vi "Initialise Notifiers and Ques.vi"(8 "error in (no error)":errorcluster) -> (0 "error out":errorcluster, 2 "Logging Queue out":refnum<queue>, 3 "Notifiers":T1)   [LabVIEW 2020]
uses:
  _Controls/Notifiers.ctl
  _Controls/Logging Queue Cluster.ctl
  _Controls/Tweezertron Ctrl Refs.ctl
  _Controls/Confocal Controls.ctl
  _Controls/iFlex.ctl
  _Controls/PIFOC Position.ctl
  _Controls/Manlight Controls.ctl
  _Controls/Exp Params.ctl
  _Controls/Image Thresholds.ctl
  _Controls/Spots.ctl
  _Controls/Spot Params.ctl
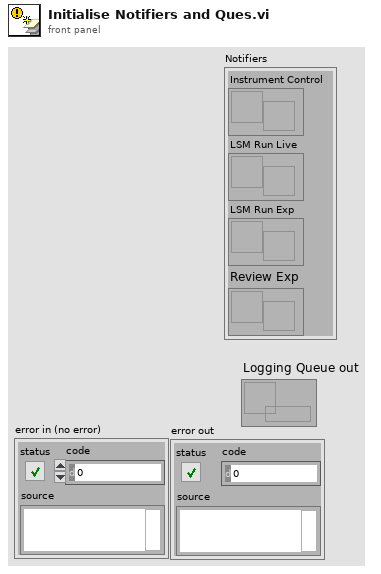
[diagram p1: front panel]
types:
  T1 = typedef "Notifiers.ctl" = cluster{"Instrument Control":refnum<notifier>, "LSM Run Live":refnum<notifier>, "LSM Run Exp":refnum<notifier>, "Review Exp":refnum<notifier>}
  T2 = typedef "Logging Queue Cluster.ctl" = cluster{"message":string, "Data for Logging":cluster{"pDataBuffer":u16[], "timestamp (ns)":u64, "PI pos (um)":dbl}, "Tweezertron Ctrl Refs":T3}
  T3 = typedef "Tweezertron Ctrl Refs.ctl" = cluster{"LSM Settings":refnum<vi>, "iFlex Control":refnum<vi>, "PIFOC Settings":refnum<vi>, "PinSelector":refnum<vi>, "Manlight Controls":refnum<vi>, "Exp Params":refnum<vi>, "Image Thresholds":refnum<vi>, "RevFrame":refnum<vi>, "Spots":refnum<vi>}
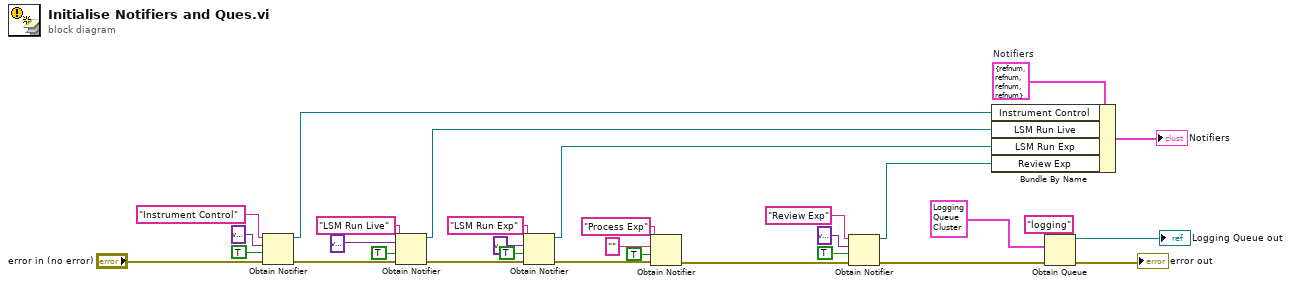
[diagram p0: block diagram]
diagram:
  w31 = T1 {"Instrument Control"=refnum, "LSM Run Live"=refnum, "LSM Run Exp"=refnum, "Review Exp"=refnum}  # Notifiers
  n1 = Obtain Notifier(name (unnamed)="Instrument Control", notification data type=variant ("element data type"), create if not found? (T)=TRUE, error in (no error)="error in (no error)") -> (notifier out=w16:refnum<notifier>, error out=w14:errorcluster)  [unwired: 1 out]
  n2 = Obtain Notifier(name (unnamed)="LSM Run Live", notification data type=variant ("element data type"), create if not found? (T)=TRUE, error in (no error)=w14) -> (notifier out=w28:refnum<notifier>, error out=w25:errorcluster)  [unwired: 1 out]
  n3 = Obtain Notifier(name (unnamed)="LSM Run Exp", notification data type=variant ("element data type"), create if not found? (T)=TRUE, error in (no error)=w25) -> (notifier out=w11:refnum<notifier>, error out=w22:errorcluster)  [unwired: 1 out]
  n4 = Obtain Notifier(name (unnamed)="Process Exp", notification data type="", create if not found? (T)=TRUE, error in (no error)=w22) -> (error out=w7:errorcluster)  [unwired: 2 out]
  n5 = Obtain Notifier(name (unnamed)="Review Exp", notification data type=variant ("element data type"), create if not found? (T)=TRUE, error in (no error)=w7) -> (notifier out=w6:refnum<notifier>, error out=w2:errorcluster)  [unwired: 1 out]
  n6 = Bundle By Name(cluster=w31, "Instrument Control"=w16, "LSM Run Live"=w28, "LSM Run Exp"=w11, "Review Exp"=w6) -> (→"Notifiers":T1)
  n7 = Obtain Queue(name (unnamed)="logging", element data type=T2 {"message"="", "Data for Logging"={"pDataBuffer"=[], "timestamp (ns)"=0, "PI pos (um)"=0.0}, "Tweezertron Ctrl Refs"={"LSM Settings"=refnum, "iFlex Control"=refnum, "PIFOC Settings"=refnum, "PinSelector"=refnum, "Manlight Controls"=refnum, "Exp Params"=refnum, "Image Thresholds"=refnum, "RevFrame"=refnum, "Spots"=refnum}} ("Logging Queue Cluster"), error in (no error)=w2) -> (queue out=→"Logging Queue out":refnum<queue>, error out=→"error out":errorcluster)  [unwired: 2 in, 1 out]
